vi "Set Terminate.vi"(8 "error in (no error)":errorcluster, 10 "Terminate":bool, 11 "Tester in":refnum<class "Tester.lvclass">) -> (0 "error out":errorcluster, 3 "Tester out":refnum<class "Tester.lvclass">)   [LabVIEW 2020]
uses:
  Tester.lvclass
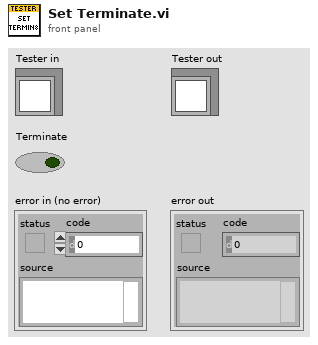
[diagram p1: front panel]
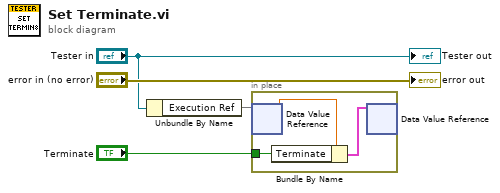
[diagram p0: block diagram]
diagram:
  n1 = Unbundle By Name("Tester in") -> ("Execution Ref"=w3)
  n2 = in-place {
    in-place-border: "Terminate" -> [w5]
    n3 = in-place-dvr #1(w3) -> (w7:dbl)  [unwired: 1 out]
    n4 = Bundle By Name(cluster=w7, "Terminate"=w5) -> (w6:cluster{})
    n5 = in-place-dvr #1(w6) -> ()  [unwired: 2 out]
  }
  "error out" <- "error in (no error)"
  "Tester out" <- "Tester in"
